vi "test 2 - normalModeCallsSysLevelMode.vi"(8 "error in (no error)":errorcluster, 11 "TestCase in":refnum<class "testcase-SyncMessage.lvclass">) -> (0 "error out":errorcluster, 3 "TestCase out":refnum<class "testcase-SyncMessage.lvclass">)   [LabVIEW 2017, in "testcase-SyncMessage.lvclass"]
uses:
  testcase-SyncMessage.lvclass
  <vilib>/addons/_JKI Toolkits/VI Tester/TestCase.llb/TestCase.lvclass
  src/user.lib/_NEVSTOP/Communicable State Machine(CSM)/Communicable State Machine.lvlib
  C:/Program Files (x86)/National Instruments/LabVIEW 2017/vi.lib/addons/_JKI Toolkits/VI Tester/TestCase.llb/TestCase.lvclass
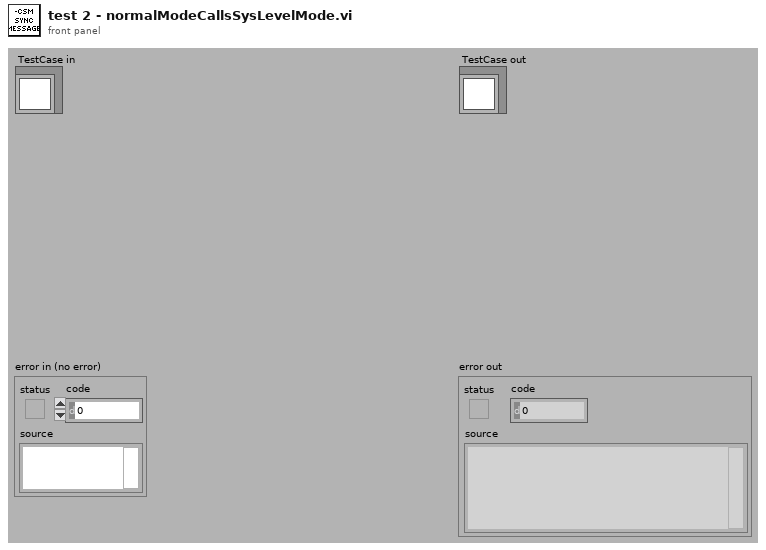
[diagram p1: front panel]
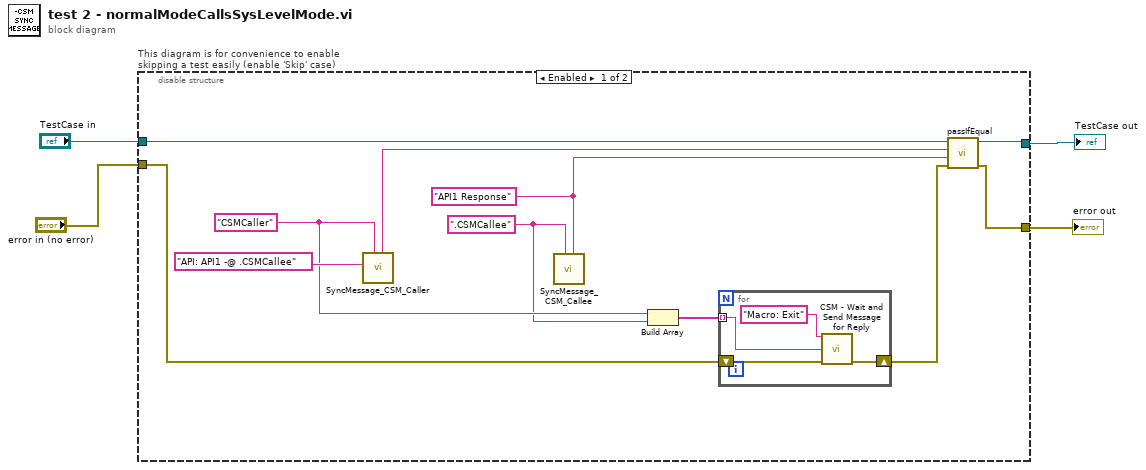
[diagram p0: block diagram]
diagram:
  n1 = disable-structure "This diagram is for convenience to enable skipping a test easily (enable 'Skip' case)" shown="Enabled" {
    disable-tunnel: "TestCase in" -> [w15 w23]
    disable-tunnel: [w14 w21] -> w2
    disable-tunnel: [w13 w22] -> w1
    disable-tunnel: "error in (no error)" -> [w12 w20]
    frame Enabled {
      w6 = ".CSMCallee" ("CSMCallee")
      w7 = "CSMCaller" ("CSMCaller")
      w9 = "API1 Response" ("API response in")
      n2 = call "SyncMessage_CSM_Caller.vi"("Name (\"\" to Use UUID)"=w7, "Intermodule Message in"="API: API1 -@ .CSMCallee") -> ("API received Response out"=w10:string)  [unwired: 9 in]
      n3 = call "SyncMessage_CSM_Callee.vi"("API response in"=w9, "Name (\"\" to Use UUID)"=w6) -> ()  [unwired: 10 in]
      n4 = Build Array(w7, w6) -> (w8:string[])
      n5 = for {
        shift-right: [w17] -> w5
        shift-left: w12 -> [w18]
        tunnel: w8 -> [w16] mode=indexing
        n6 = call "CSM - Wait and Send Message for Reply.vi"("State"="Macro: Exit", "Target Module"=w16, "Error In (No Error)"=w18) -> ("error out"=w17:errorcluster)  [unwired: 10 in, 2 out]
      }
      n7 = call-dynamic "passIfEqual.vi"("error in (no error)"=w5, "y"=w9, "x"=w10, "TestCase in"=w15) -> ("error out"=w13:errorcluster, "TestCase out"=w14:refnum<class "testcase-SyncMessage.lvclass">)  [unwired: 6 in]
    }
    frame Disabled {
      # "skip test result while test is under development"
      n8 = call <vilib>:"skip.vi"("error in (no error)"=w20, "TestCase in"=w23) -> ("error out"=w22:errorcluster, "TestCase out"=w21:refnum<class "testcase-SyncMessage.lvclass">)  [unwired: 8 in]
    }
  }
  "error out" <- w1
  "TestCase out" <- w2
